vi "CRYGet HZ Input Shortcut Menu.vi"(11 "Runtime Menu Ref In":refnum<k9>) -> (0 "error out":errorcluster, 3 "Runtime Menu Ref Out":refnum<k9>)   [LabVIEW 2013]
uses:
  CRYMainGlobal.vi
panel:
  out "Item tag":string[](array[string])=["USER_INPUT", "CURVE_VALUE"]
  out "Item Name":string[](array[string])
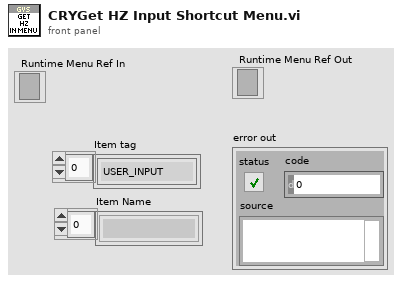
[diagram p1: front panel]
types:
  T1 = enum32{"English", "Chinese", "Korean", "Japanese", "Russian", "Chinese traditional"}
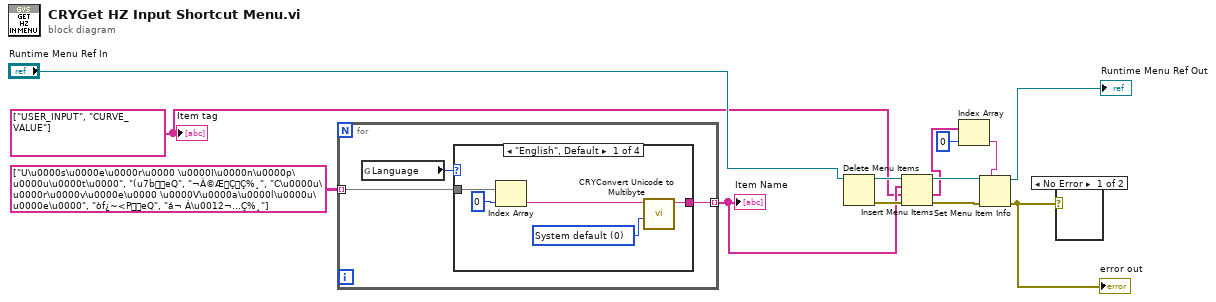
[diagram p0: block diagram]
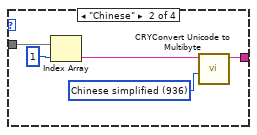
[diagram p3: hidden frame]
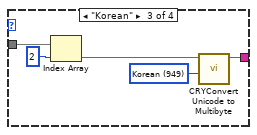
[diagram p4: hidden frame]
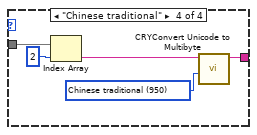
[diagram p5: hidden frame]
diagram:
  w1 = string[] ["USER_INPUT", "CURVE_VALUE"]
  n1 = for {
    tunnel: string[][] [["U\u0000s\u0000e\u0000r\u0000 \u0000I\u0000n\u0000p\u0000u\u0000t\u0000", "(u7beQ", "¬À©ÆÇÇ%¸"], ["C\u0000u\u0000r\u0000v\u0000e\u0000 \u0000V\u0000a\u0000l\u0000u\u0000e\u0000", "òf¿~<PeQ", "á¬ Á\u0012¬…Ç%¸"]] -> [w15] mode=indexing
    tunnel: [w14] -> w2 mode=indexing
    n2 = global read "CRYMainGlobal.vi" "Language"() -> (w16:T1)
    n3 = case shown="\"English\", Default" w16 {
      tunnel: w15 -> [w21 w24 w28 w33]
      tunnel: [w17 w23 w30 w35] -> w14
      frame "English", Default {
        w18 = 0 items=["System default"=0, "Latin-1"=1252, "Japanese"=932, "Korean"=947, "Chinese simplified"=936, "Chinese traditional"=950, "Central Europe"=1250, "Cyrillic"=1251, "Greek"=1253, "Turkish"=1254, "Hebrew"=1255, "Arabic"=1256, "Baltic"=1257, "Thai"=874, "Vietnamese"=783, "UTF8"=65001, "UTF-7"=65000] ("Code Page")
        n4 = Index Array(array=w21, index=0) -> (element=w19:string)
        n5 = call "CRYConvert Unicode to Multibyte.vi"("Code Page"=w18, "Unicode String"=w19) -> ("Multibyte string"=w17:string)  [unwired: 8 in, 1 out]
      }
      frame "Chinese" {
        w25 = 936 items=["System default"=0, "Latin-1"=1252, "Japanese"=932, "Korean"=947, "Chinese simplified"=936, "Chinese traditional"=950, "Central Europe"=1250, "Cyrillic"=1251, "Greek"=1253, "Turkish"=1254, "Hebrew"=1255, "Arabic"=1256, "Baltic"=1257, "Thai"=874, "Vietnamese"=783, "UTF8"=65001, "UTF-7"=65000] ("Code Page")
        n6 = Index Array(array=w24, index=1) -> (element=w22:string)
        n7 = call "CRYConvert Unicode to Multibyte.vi"("Code Page"=w25, "Unicode String"=w22) -> ("Multibyte string"=w23:string)  [unwired: 8 in, 1 out]
      }
      frame "Korean" {
        w27 = 949 items=["System default"=0, "Latin-1"=1252, "Japanese"=932, "Korean"=949, "Chinese simplified"=936, "Chinese traditional"=950, "Central Europe"=1250, "Cyrillic"=1251, "Greek"=1253, "Turkish"=1254, "Hebrew"=1255, "Arabic"=1256, "Baltic"=1257, "Thai"=874, "Vietnamese"=783, "UTF8"=65001, "UTF-7"=65000] ("Code Page")
        n8 = Index Array(array=w28, index=2) -> (element=w29:string)
        n9 = call "CRYConvert Unicode to Multibyte.vi"("Code Page"=w27, "Unicode String"=w29) -> ("Multibyte string"=w30:string)  [unwired: 8 in, 1 out]
      }
      frame "Chinese traditional" {
        w32 = 950 items=["System default"=0, "Latin-1"=1252, "Japanese"=932, "Korean"=949, "Chinese simplified"=936, "Chinese traditional"=950, "Central Europe"=1250, "Cyrillic"=1251, "Greek"=1253, "Turkish"=1254, "Hebrew"=1255, "Arabic"=1256, "Baltic"=1257, "Thai"=874, "Vietnamese"=783, "UTF8"=65001, "UTF-7"=65000] ("Code Page")
        n10 = Index Array(array=w33, index=2) -> (element=w34:string)
        n11 = call "CRYConvert Unicode to Multibyte.vi"("Code Page"=w32, "Unicode String"=w34) -> ("Multibyte string"=w35:string)  [unwired: 8 in, 1 out]
      }
    }
  }
  "Item Name" <- w2
  n12 = Delete Menu Items(9:"Runtime Menu Ref In") -> (0:w6:errorcluster, 3:w12:refnum<k9>)  [unwired: 2 in, 1 out]
  n13 = Insert Menu Items(6:w6, 7:w1, 8:w2, 9:w12) -> (0:w7:errorcluster, 1:w9:string[], 3:w11:refnum<k9>)  [unwired: 2 out]
  n14 = Index Array(array=w9, index=0) -> (element=w8:string)
  n15 = Set Menu Item Info(7:w8, 8:w7, 11:w11) -> (0:w5:errorcluster, 3:→"Runtime Menu Ref Out":refnum<k9>)  [unwired: 3 in, 1 out]
  "error out" <- w5
  n16 = case shown="No Error" w5 {
    frame No Error {
    }
    frame Error {
    }
  }
  "Item tag" <- w1
